vi "FdxCmdTMSetTSListCvi.vi"(6 "NumberofSubscribers":u16, 7 "TSListDataPtr":u32, 8 "error in":errorcluster, 9 "RequestNumber":u16, 10 "TMHandle":u32, 11 "InstrumentHandle":u32) -> (0 "error out":errorcluster, 2 "TMHandleOut":u32, 3 "InstrumentHandle":u32)   [LabVIEW 2020, in "AIM664LV.lvlib"]
doc: "This function is used to set up a Time Manager for communication with a subscriber. This function can not be called once a Time Manager has been started."
uses:
  AIM664LV.lvlib
  AFDX_LibraryAdmin/FdxGlobalDllPath.vi
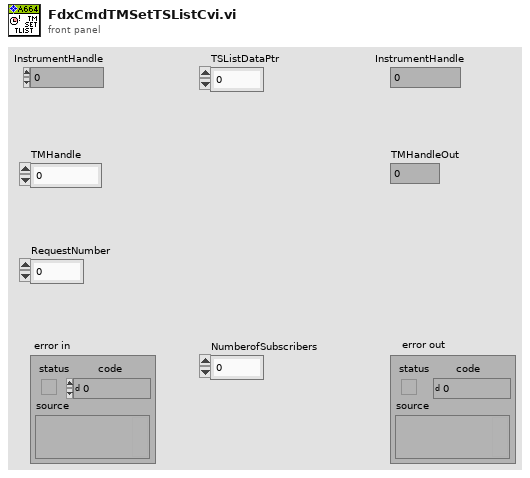
[diagram p1: front panel]
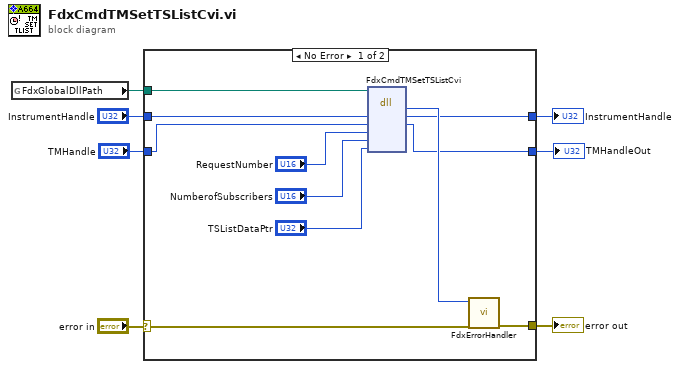
[diagram p0: block diagram]
diagram:
  n1 = global read "FdxGlobalDllPath.vi" "FdxGlobalDllPath"() -> (w5:path)
  n2 = case shown="No Error" "error in" {
    selector: "error in" -> [w17 w21]
    tunnel: [w18 w21] -> w7
    tunnel: w5 -> [w12 _]
    tunnel: "InstrumentHandle" -> [w11 w20]
    tunnel: [w10 w20] -> w3
    tunnel: [w9 w19] -> w2
    tunnel: "TMHandle" -> [w8 w19]
    frame No Error {
      n3 = dll-call lib="aim_fdx.19.dll" fn="FdxCmdTMSetTSListCvi"(path in=w12, "InstrumentHandle"=w11, "TMHandle"=w8, "RequestNumber"="RequestNumber", "NumberofSubscribers"="NumberofSubscribers", "TSListData"="TSListDataPtr") -> ("status"=w16:i32, "InstrumentHandle"=w10:u32, "TMHandle"=w9:u32)  [unwired: 5 in, 2 out]
      n4 = call "FdxErrorHandler.vi"("error in"=w17, "AIM Error"=w16) -> ("error out"=w18:errorcluster)  [unwired: 9 in]
    }
    frame Error {
    }
  }
  "error out" <- w7
  "InstrumentHandle" <- w3
  "TMHandleOut" <- w2
